vi "solar_excel Worksheet Parse (tsv).vi"(10 "Remove Quotes? (F)":bool, 11 "Tab Delimited String":string) -> (2 "Worksheets Cells":cluster{"Cells":string[][]}[](array[cluster]), 3 "Worksheets":string[](array[string]))   [LabVIEW 2018]
doc: "This parses a tab delimited text file (*.tsv) into Worksheets specified by sections (i.e. '[MySheet1]')\n\n[MySheet1] -> Creates 'MySheet1'\nA\\tB\\tC\nD\\tE\\tF\n[MySheet2] -> Creates 'MySheet2'\n1\\t2\\t3\n4\\t5\\t6"
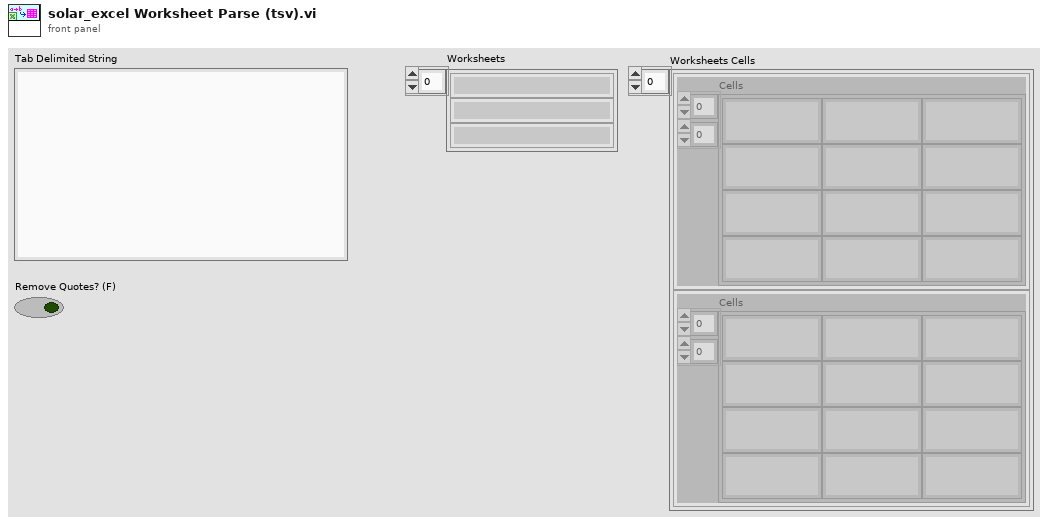
[diagram p1: front panel]
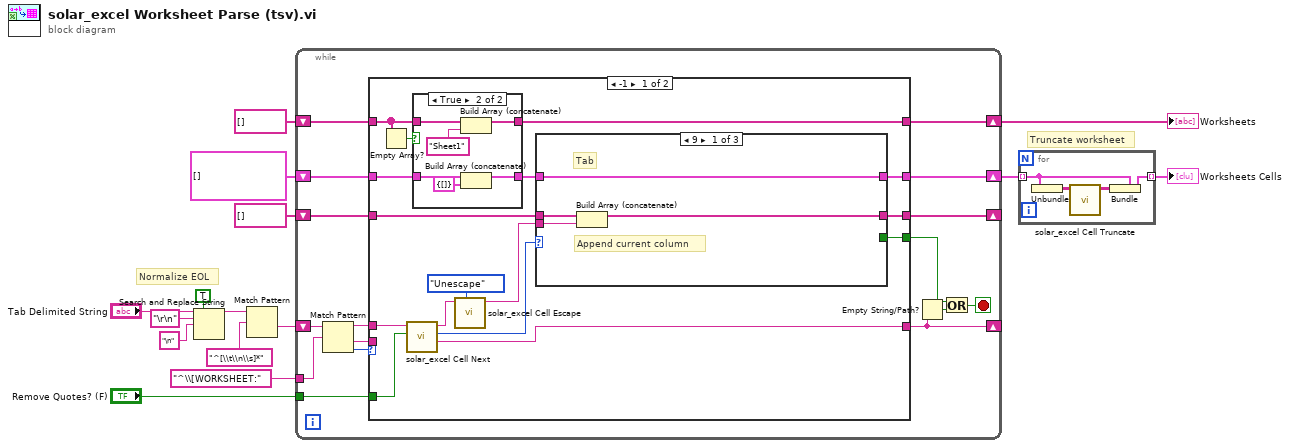
[diagram p0: block diagram]
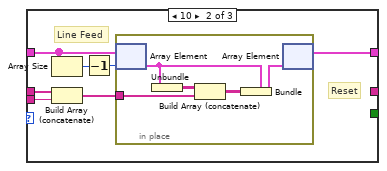
[diagram p3: hidden frame]
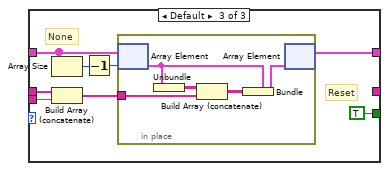
[diagram p4: hidden frame]
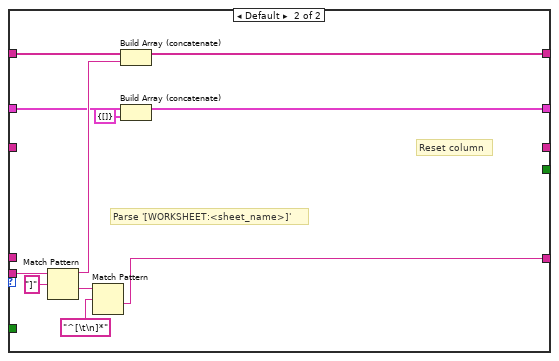
[diagram p5: hidden frame]
diagram:
  # "Truncate worksheet"
  # "Normalize EOL"
  n1 = Search and Replace String(replace all?=TRUE ("replace all? (F)"), input string="Tab Delimited String", search string="\r\n", replace string="\n" ("search string")) -> (result string=w1:string)  [unwired: 4 in, 3 out]
  n2 = Match Pattern(string=w1, regular expression="^[\\t\\n\\s]*") -> (after substring=w15:string)  [unwired: 1 in, 3 out]
  n3 = while {
    shift-right: [w19] -> _
    shift-left: w15 -> [w29]
    shift-right: [w28] -> w13
    shift-left: string[] [] ("Worksheets") -> [w27]
    shift-right: [w26] -> w3
    shift-left: cluster{"Cells":string[][]}[] [] ("Worksheets Cells") -> [w25]
    shift-right: [w21] -> _
    shift-left: string[] [] ("Cells") -> [w22]
    tunnel: "^\\[WORKSHEET:" ("regular expression") -> [w20]
    tunnel: "Remove Quotes? (F)" -> [w16]
    stop <- w18 stop-if-true
    n4 = Match Pattern(string=w29, regular expression=w20) -> (before substring=w24:string, after substring=w30:string, offset past match=w31:i32)  [unwired: 1 in, 1 out]
    n5 = case shown="-1" w31 {
      tunnel: w30 -> [_ w94]
      tunnel: [w41 w92] -> w28
      tunnel: w27 -> [w40 w93]
      tunnel: [w36 w88] -> w19
      tunnel: [w44 w86] -> w26
      tunnel: w25 -> [w38 w87]
      tunnel: w24 -> [w47 _]
      tunnel: [w42 _] -> w23
      tunnel: w22 -> [w43 _]
      tunnel: [w45 _] -> w21
      tunnel: w16 -> [w35 _]
      frame -1 {
        n6 = Empty Array?(array=w40) -> (empty?=w37:bool)
        n7 = call "solar_excel Cell Next.vi"("Remove Quotes? (F)"=w35, "Tab Delimited String in"=w47) -> ("Remaining"=w36:string, "Delimiter"=w46:u8, "Cell out"=w33:string)  [unwired: 6 in, 1 out]
        n8 = case shown="True" w37 {
          tunnel: [w49 w53] -> w41
          tunnel: w40 -> [w49 w55]
          tunnel: [w48 w51] -> w39
          tunnel: w38 -> [w48 w54]
          frame False {
          }
          frame True {
            n9 = Build Array (concatenate)(w55, "Sheet1") -> (w53:string[])
            n10 = Build Array (concatenate)(w54, cluster{"Cells":string[][]} {"Cells"=[]} ("Worksheet Data")) -> (w51:cluster{"Cells":string[][]}[])
          }
        }
        n11 = call "solar_excel Cell Escape.vi"("Action (Escape)"=enum8{"Escape", "Unescape"}."Unescape", "String in"=w33) -> ("String out"=w32:string)  [unwired: 9 in]
        n12 = case shown="9" w46 {
          tunnel: w43 -> [w58 w63 w76]
          tunnel: [w57 _ _] -> w45
          tunnel: [w59 w62 w75] -> w44
          tunnel: w39 -> [w59 w65 w78]
          tunnel: w32 -> [w56 w60 w73]
          tunnel: [_ _ TRUE] -> w42
          frame 9 {
            # "Tab"
            # "Append current column"
            n13 = Build Array (concatenate)(w58, w56) -> (w57:string[])
          }
          frame 10 {
            # "Reset"
            # "Line Feed"
            n14 = Array Size(array=w65) -> (size(s)=w66:i32)
            n15 = Build Array (concatenate)(w63, w60) -> (w61:string[])
            n16 = Decrement(x=w66) -> (x-1=w64:i32)
            n17 = in-place {
              in-place-border: w61 -> [w68]
              n18 = in-place-array #1(w65, w64) -> (w71:cluster{"Cells":string[][]})
              n19 = Unbundle(w71) -> ("Cells"=w69:string[][])
              n20 = Build Array (concatenate)(w69, w68) -> (w67:string[][])
              n21 = Bundle(cluster=w71, "Cells"=w67) -> (w70:cluster{"Cells":string[][]})
              n22 = in-place-array #1(w70) -> (w62:cluster{"Cells":string[][]}[])  [unwired: 1 out]
            }
          }
          frame Default {
            # "Reset"
            # "None"
            n23 = Array Size(array=w78) -> (size(s)=w79:i32)
            n24 = Build Array (concatenate)(w76, w73) -> (w74:string[])
            n25 = Decrement(x=w79) -> (x-1=w77:i32)
            n26 = in-place {
              in-place-border: w74 -> [w81]
              n27 = in-place-array #2(w78, w77) -> (w84:cluster{"Cells":string[][]})
              n28 = Unbundle(w84) -> ("Cells"=w82:string[][])
              n29 = Build Array (concatenate)(w82, w81) -> (w80:string[][])
              n30 = Bundle(cluster=w84, "Cells"=w80) -> (w83:cluster{"Cells":string[][]})
              n31 = in-place-array #2(w83) -> (w75:cluster{"Cells":string[][]}[])  [unwired: 1 out]
            }
          }
        }
      }
      frame Default {
        # "Parse '[WORKSHEET:<sheet_name>]'"
        # "Reset column"
        n32 = Match Pattern(string=w94, regular expression="]") -> (before substring=w91:string, after substring=w89:string)  [unwired: 1 in, 2 out]
        n33 = Match Pattern(string=w89, regular expression="^[\t\n]*") -> (after substring=w88:string)  [unwired: 1 in, 3 out]
        n34 = Build Array (concatenate)(w93, w91) -> (w92:string[])
        n35 = Build Array (concatenate)(w87, cluster{"Cells":string[][]} {"Cells"=[]} ("Worksheet Data")) -> (w86:cluster{"Cells":string[][]}[])
      }
    }
    n36 = Empty String/Path?(string/path=w19) -> (empty?=w17:bool)
    n37 = Or(x=w23, y=w17) -> (x .or. y?=w18:bool)
  }
  "Worksheets" <- w13
  n38 = for {
    tunnel: [w98] -> w4 mode=indexing
    tunnel: w3 -> [w99] mode=indexing
    n39 = Unbundle(w99) -> ("Cells"=w97:string[][])
    n40 = call "solar_excel Cell Truncate.vi"("Cells in"=w97) -> ("Truncated Cells out"=w96:string[][])  [unwired: 10 in]
    n41 = Bundle(cluster=w99, "Cells"=w96) -> (w98:cluster{"Cells":string[][]})
  }
  "Worksheets Cells" <- w4
